vi "Get_Angular_Position.vi"(8 "error in (no error)":errorcluster) -> (0 "error out":errorcluster, 2 "AngularPosition":T1)   [LabVIEW 2019]
uses:
  <vilib>/Utility/error.llb/Error Cluster From Error Code.vi
  <vilib>/ErrorRing/Error Ring.xnode
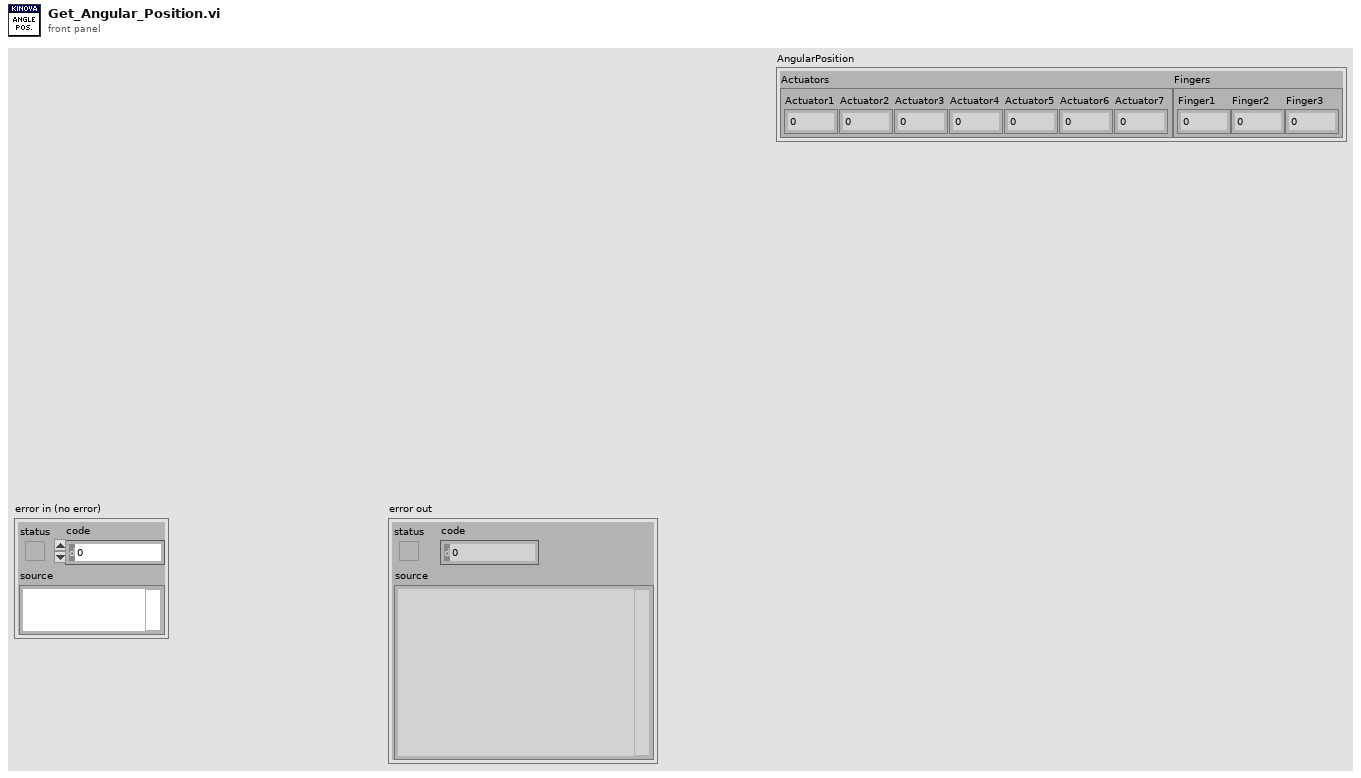
[diagram p1: front panel]
types:
  T1 = cluster{"Actuators":cluster{"Actuator1":sgl, "Actuator2":sgl, "Actuator3":sgl, "Actuator4":sgl, "Actuator5":sgl, "Actuator6":sgl, "Actuator7":sgl}, "Fingers":cluster{"Finger1":sgl, "Finger2":sgl, "Finger3":sgl}}
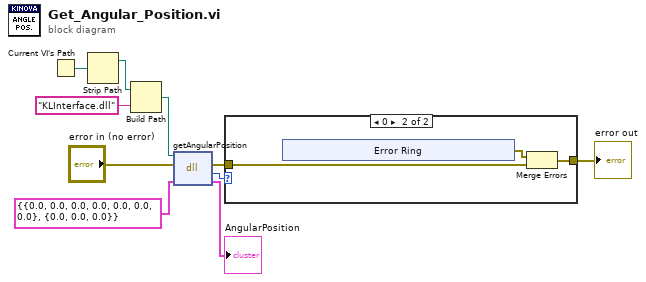
[diagram p0: block diagram]
diagram:
  n1 = Current VI's Path() -> (path=w7:path)
  n2 = Strip Path(path=w7) -> (stripped path=w6:path)  [unwired: 1 out]
  n3 = Build Path(base path=w6, name or relative path="KLInterface.dll") -> (appended path=w1:path)
  n4 = dll-call lib="C:/Users/mcjssdcc/source/repos/Kinova Labview Interface/Debug/KLInterface.dll" fn="getAngularPosition"(path in=w1, error in="error in (no error)", "actuators"=T1 {"Actuators"={"Actuator1"=0.0, "Actuator2"=0.0, "Actuator3"=0.0, "Actuator4"=0.0, "Actuator5"=0.0, "Actuator6"=0.0, "Actuator7"=0.0}, "Fingers"={"Finger1"=0.0, "Finger2"=0.0, "Finger3"=0.0}} ("AngularPosition")) -> (error out=w9:errorcluster, "return type"=w8:i32, "actuators"=→"AngularPosition":T1)  [unwired: 1 in, 1 out]
  n5 = case shown="0" w8 {
    tunnel: [w11 w13] -> w5
    tunnel: w9 -> [w11 w12]
    frame 1, Default {
    }
    frame 0 {
      n6 = xnode "Error Ring"() -> ("error out"=w14:errorcluster)
      n7 = Merge Errors(w14, w12) -> (w13:errorcluster)
    }
  }
  "error out" <- w5
